vi "Make_Competion_For_Elongations_101_Points-1.vi"(4 "error IN":errorcluster, 7 "[IN] Subtracks in Row":T1(array[cluster])) -> (0 "error OUT":errorcluster, 3 "[OUT Subtracks in Row":T1(array[cluster]))   [LabVIEW 2017]
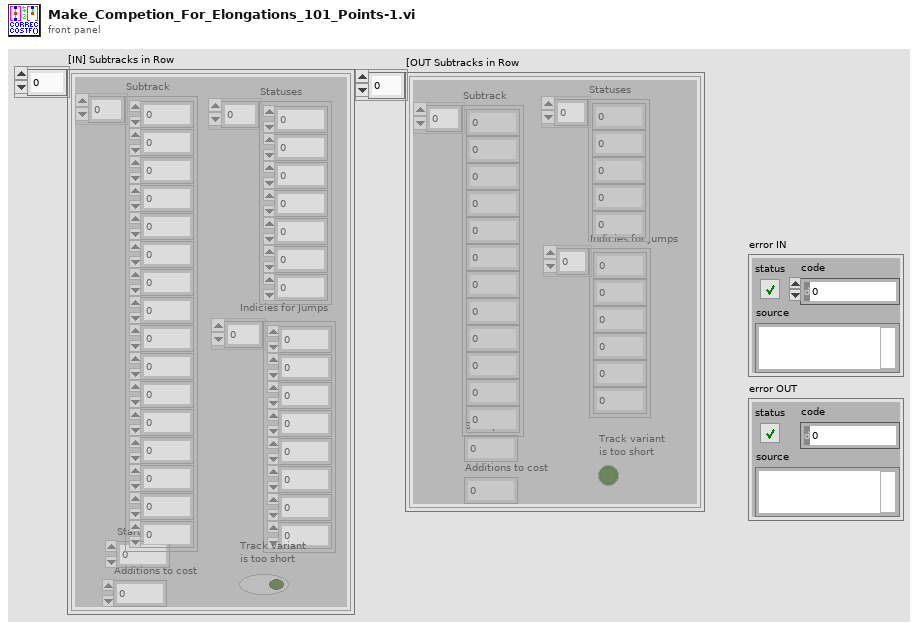
[diagram p1: front panel]
types:
  T1 = cluster{"Subtrack":dbl[], "Statuses":i16[], "Start pos":i32, "Additions to cost":i8, "Track variant \nis too short":bool, "Indicies for Jumps":i32[]}[]
  T2 = cluster{"Subtrack":dbl[], "Statuses":i16[], "Start pos":i32, "Additions to cost":i8, "Track variant \nis too short":bool, "Indicies for Jumps":i32[]}
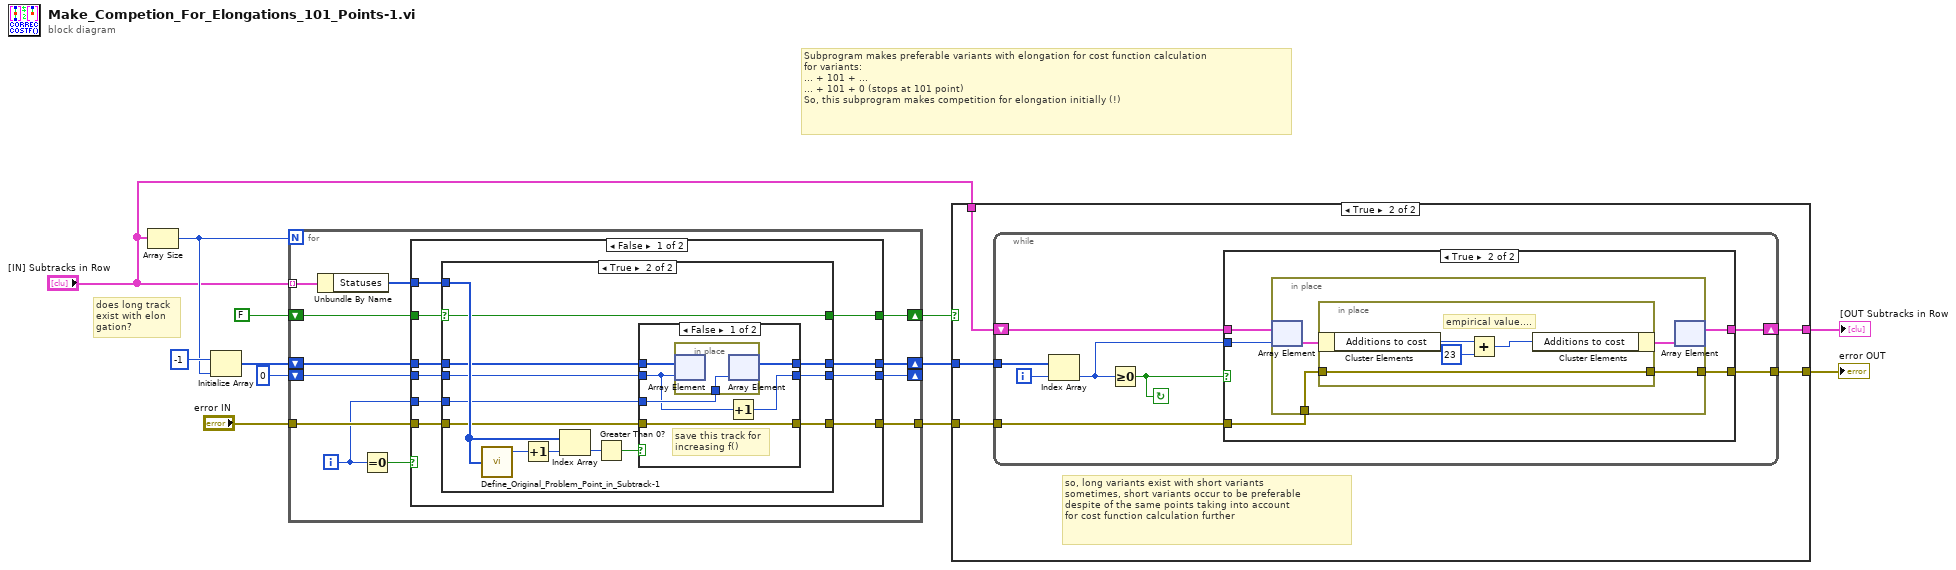
[diagram p0: block diagram]
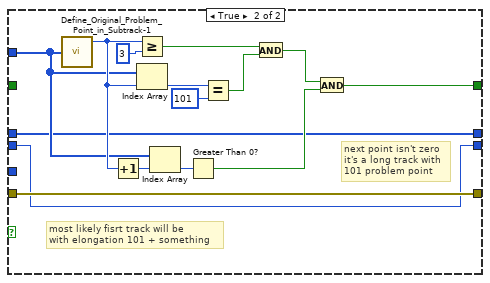
[diagram p6: hidden frame]
diagram:
  # "Subprogram makes preferable variants with elongation for cost function calculation\nfor variants: \n... + 101 + ... \n... + 101 + 0 (stops at 101 point) \nSo, this subprogram makes competition for elongation initially (!)"
  # "does long track \nexist with elon\ngation?"
  n1 = Array Size(array="[IN] Subtracks in Row") -> (size(s)=w10:i32)
  n2 = Initialize Array(-1 ("element"), w10) -> (w9:i32[])
  n3 = for {
    N: w10 -> [_]
    tunnel: "[IN] Subtracks in Row" -> [w24] mode=indexing
    shift-right: [w17] -> w7
    shift-left: FALSE -> [w16]
    shift-right: [w19] -> w4
    shift-left: w9 -> [w20]
    tunnel: "error IN" -> [w21]
    tunnel: [w18] -> w5
    shift-right: [w13] -> _
    shift-left: 0 -> [w15]
    i -> [w14]
    n4 = Unbundle By Name(w24) -> ("Statuses"=w22:i16[])
    n5 = Equal To 0?(x=w14) -> (x = 0?=w23:bool)
    n6 = case shown="False" w23 {
      tunnel: w22 -> [w32 w72]
      tunnel: w21 -> [w31 w64]
      tunnel: w20 -> [w30 w65]
      tunnel: [w27 w65] -> w19
      tunnel: [w25 w64] -> w18
      tunnel: [w33 w63] -> w17
      tunnel: w16 -> [w34 _]
      tunnel: w15 -> [w29 w62]
      tunnel: w14 -> [w28 _]
      tunnel: [w26 w62] -> w13
      frame False {
        n7 = case shown="True" w34 {
          selector: w34 -> [w38 w42]
          tunnel: [w38 w42] -> w33
          tunnel: w32 -> [_ w48]
          tunnel: w31 -> [w35 w40]
          tunnel: w30 -> [w37 w46]
          tunnel: w29 -> [w36 w45]
          tunnel: w28 -> [_ w44]
          tunnel: [w37 w43] -> w27
          tunnel: [w36 w41] -> w26
          tunnel: [w35 w39] -> w25
          frame False {
          }
          frame True {
            n8 = call "Define_Original_Problem_Point_in_Subtrack-1.vi"("[IN] Statuses"=w48) -> ("[OUT] Index of Problem Point\nin Subtrack (Original)"=w50:i32)  [unwired: 3 in, 1 out]
            n9 = Increment(x=w50) -> (x+1=w51:i32)
            n10 = Index Array(array=w48, index=w51) -> (element=w49:i16)
            n11 = Greater Than 0?(x=w49) -> (x > 0?=w47:bool)
            n12 = case shown="False" w47 {
              tunnel: w46 -> [w57 w61]
              tunnel: w45 -> [w54 w60]
              tunnel: w44 -> [w56 _]
              tunnel: [w55 w61] -> w43
              tunnel: [w53 w60] -> w41
              tunnel: w40 -> [w52 w59]
              tunnel: [w52 w59] -> w39
              frame False {
                # "save this track for \nincreasing f()"
                n13 = in-place {
                  in-place-border: w56 -> [w58]
                  n14 = in-place-array #1(w57, w54) -> ()  [unwired: 1 out]
                  n15 = in-place-array #1(w58) -> (w55:i32[])  [unwired: 1 out]
                }
                n16 = Increment(x=w54) -> (x+1=w53:i32)
              }
              frame True {
              }
            }
          }
        }
      }
      frame True {
        # "next point isn't zero\nit's a long track with\n101 problem point"
        # "most likely fisrt track will be \nwith elongation 101 + something"
        n17 = call "Define_Original_Problem_Point_in_Subtrack-1.vi"("[IN] Statuses"=w72) -> ("[OUT] Index of Problem Point\nin Subtrack (Original)"=w73:i32)  [unwired: 3 in, 1 out]
        n18 = Increment(x=w73) -> (x+1=w71:i32)
        n19 = Greater Or Equal?(x=w73, y=3) -> (x >= y?=w69:bool)
        n20 = Index Array(array=w72, index=w73) -> (element=w75:i16)
        n21 = Index Array(array=w72, index=w71) -> (element=w70:i16)
        n22 = Greater Than 0?(x=w70) -> (x > 0?=w66:bool)
        n23 = Equal?(x=w75, y=i16 101) -> (x = y?=w68:bool)
        n24 = And(x=w69, y=w68) -> (x .and. y?=w67:bool)
        n25 = And(x=w67, y=w66) -> (x .and. y?=w63:bool)
      }
    }
  }
  n26 = case shown="True" w7 {
    tunnel: "[IN] Subtracks in Row" -> [w77 w81]
    tunnel: w5 -> [w78 w83]
    tunnel: w4 -> [_ w82]
    tunnel: [w78 w80] -> w3
    tunnel: [w77 w79] -> w2
    frame False {
    }
    frame True {
      # "so, long variants exist with short variants\nsometimes, short variants occur to be preferable\ndespite of the same points taking into account \nfor cost function calculation further"
      n27 = while {
        tunnel: w83 -> [w85]
        tunnel: w82 -> [w91]
        shift-right: [w86] -> w79
        shift-left: w81 -> [w89]
        tunnel: [w84] -> w80
        i -> [w90]
        stop <- w87 continue-if-true
        n28 = Index Array(array=w91, index=w90) -> (element=w88:i32)
        n29 = Greater Or Equal To 0?(x=w88) -> (x >= 0?=w87:bool)
        n30 = case shown="True" w87 {
          tunnel: w89 -> [w93 w98]
          tunnel: w88 -> [_ w97]
          tunnel: [w93 w95] -> w86
          tunnel: w85 -> [w92 w96]
          tunnel: [w92 w94] -> w84
          frame False {
          }
          frame True {
            n31 = in-place {
              in-place-border: w96 -> [w101]
              in-place-border: [w99] -> w94
              n32 = in-place-array #2(w98, w97) -> (w102:T2)
              n33 = in-place {
                in-place-border: w101 -> [w103]
                in-place-border: [w103] -> w99
                # "empirical value...."
                n34 = in-place-cluster #3(w102) -> ("Additions to cost"=w106:i8)
                n35 = Add(x=w106, y=i8 23) -> (x+y=w105:i8)
                n36 = in-place-cluster #3("Additions to cost"=w105) -> (w100:T2)
              }
              n37 = in-place-array #2(w100) -> (w95:T1)  [unwired: 1 out]
            }
          }
        }
      }
    }
  }
  "error OUT" <- w3
  "[OUT Subtracks in Row" <- w2
